vi "decodeInt8.vi"(8 "error in (no error)":errorcluster, 11 "ByteArray":u8[](array[numeric]) format="%x") -> (0 "error out":errorcluster, 1 "Int8":i8, 2 "Variant":variant, 3 "RemainingBytes":u8[](array[numeric]) format="%x", 5 "Type":string)   [LabVIEW 2015, in "MsgPack.lvlib"]
uses:
  MsgPack.lvlib
  <vilib>/ErrorRing/Error Ring.xnode
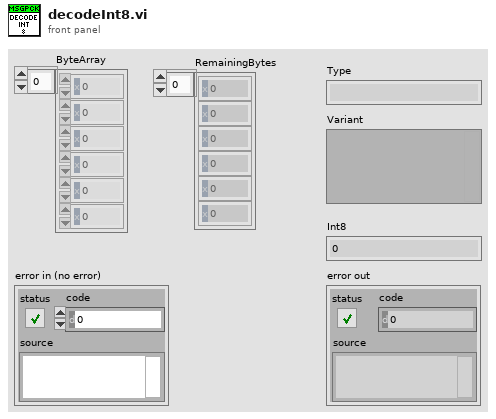
[diagram p1: front panel]
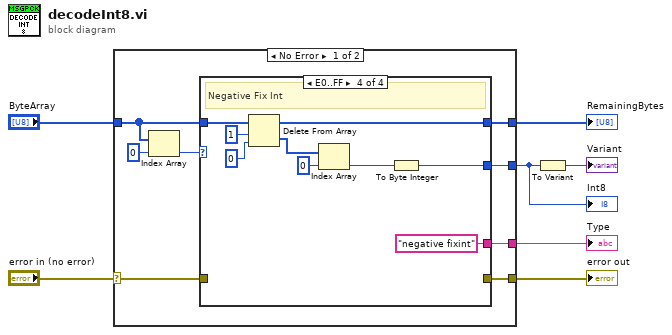
[diagram p0: block diagram]
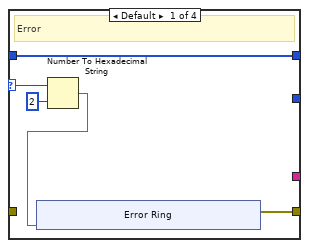
[diagram p2: hidden frame]
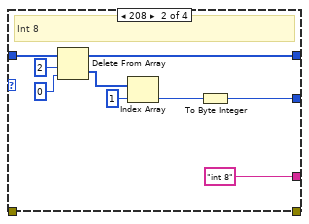
[diagram p3: hidden frame]
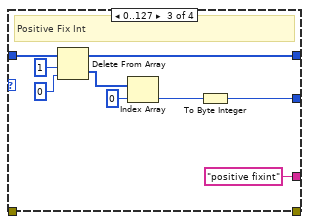
[diagram p4: hidden frame]
diagram:
  n1 = case shown="No Error" "error in (no error)" {
    selector: "error in (no error)" -> [w12 w54]
    tunnel: [w15 w54] -> w6
    tunnel: [w14 _] -> w5
    tunnel: [w13 _] -> w4
    tunnel: "ByteArray" -> [w10 w53]
    tunnel: [w11 w53] -> w2
    frame No Error {
      n2 = Index Array(array=w10, index=0) -> (element=w9:u8)
      n3 = case shown="E0..FF" w9 {
        selector: w9 -> [w17 _ _ _]
        tunnel: [w19 _ _ _] -> w15
        tunnel: w12 -> [_ _ _ _]
        tunnel: [_ "int 8" "positive fixint" "negative fixint"] -> w14
        tunnel: [_ w26 w35 w44] -> w13
        tunnel: [w20 w31 w40 w49] -> w11
        tunnel: w10 -> [w20 w32 w41 w50]
        frame Default {
          # "Error"
          n4 = Number To Hexadecimal String(1:i16 2 ("width (-)"), 2:w17) -> (0:w16:string)
          n5 = xnode "Error Ring"("parameter 0"=w16) -> ("error out"=w19:errorcluster)
        }
        frame 208 {
          # "Int 8"
          n6 = Delete From Array(array=w32, length=2, index=0) -> (deleted portion=w29:u8[], array with subset deleted=w31:u8[])
          n7 = Index Array(array=w29, index=1) -> (element=w27:u8)
          n8 = To Byte Integer(number=w27) -> (8bit integer=w26:i8)
        }
        frame 0..127 {
          # "Positive Fix Int"
          n9 = Delete From Array(array=w41, length=1, index=0) -> (deleted portion=w38:u8[], array with subset deleted=w40:u8[])
          n10 = Index Array(array=w38, index=0) -> (element=w36:u8)
          n11 = To Byte Integer(number=w36) -> (8bit integer=w35:i8)
        }
        frame 224..255 {
          # "Negative Fix Int"
          n12 = Delete From Array(array=w50, length=1, index=0) -> (deleted portion=w47:u8[], array with subset deleted=w49:u8[])
          n13 = Index Array(array=w47, index=0) -> (element=w45:u8)
          n14 = To Byte Integer(number=w45) -> (8bit integer=w44:i8)
        }
      }
    }
    frame Error {
    }
  }
  "error out" <- w6
  "Type" <- w5
  "Int8" <- w4
  "RemainingBytes" <- w2
  n15 = To Variant(anything=w4) -> (Variant=→"Variant":variant)
